vi "MEMR-Compute Noise Floor (single traces).vi"(0 "State In":T2, 5 "Analysis":T1, 7 "Avg":dbl[][](array[numeric]), 9 "Navg":i32, 11 "N":i32=1000) -> (4 "Noise spectra":cluster{"Freq (Hz)":dbl[], "Mag (dB)":dbl[]}[](array[cluster]))   [LabVIEW 2020]
uses:
  Typedefs/MEMR-Analysis State.ctl
  MEMR-Offline Analysis Parameters.ctl
  Typedefs/MEMR-Analysis.ctl
  PXI DAQ VIs/Utility VIs/Array Dimensions (2D).vi
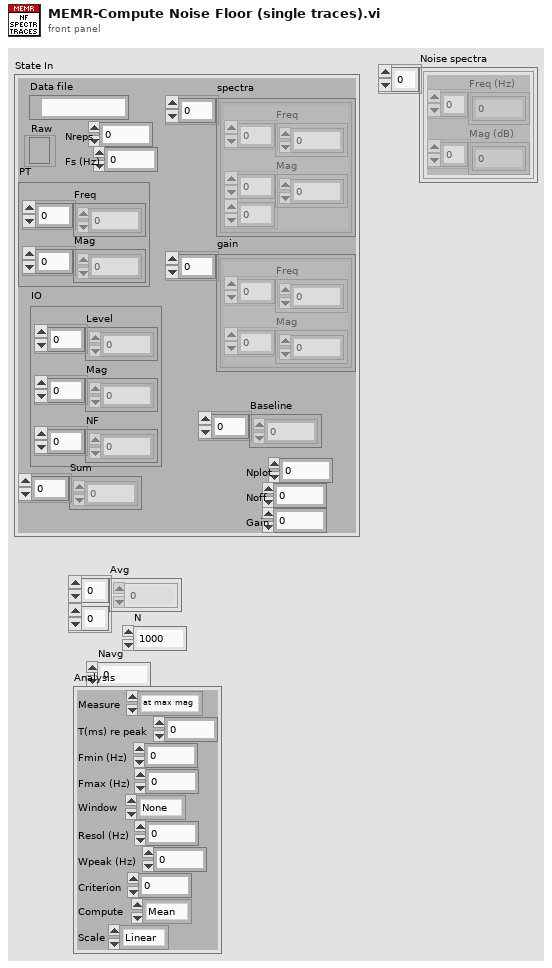
[diagram p1: front panel]
types:
  T1 = typedef "MEMR-Offline Analysis Parameters.ctl" = cluster{"Measure":enum16{"at max mag", "at max gain", "over window", "optimize", "Keefe"}, "T(ms) re peak":dbl, "Fmin (Hz)":dbl, "Fmax (Hz)":dbl, "Window":enum16{"None", "Hanning", "Hamming"}, "Resol (Hz)":dbl, "Wpeak (Hz)":dbl, "Criterion":dbl, "Compute":enum16{"Mean", "Sum"}, "Scale":enum16{"Linear", "Log"}}
  T2 = typedef "MEMR-Analysis State.ctl" = cluster{"Data file":path, "Raw":refnum<file>, "PT":cluster{"Freq":dbl[], "Mag":dbl[]}, "IO":cluster{"Level":dbl[], "Mag":dbl[], "NF":dbl[]}, "Nreps":i32, "Fs (Hz)":dbl, "Sum":dbl[], "Nplot":i32, "Noff":i32, "Gain":dbl, "spectra":cluster{"Freq":dbl[], "Mag":dbl[][]}[], "gain":cluster{"Freq":dbl[], "Mag":dbl[]}[], "Baseline":dbl[]}
  T3 = typedef "MEMR-Analysis.ctl" = cluster{"T(ms) re peak":dbl, "Fmin (Hz)":dbl, "Fmax (Hz)":dbl, "Window":enum16{"None", "Hanning", "Hamming"}, "Gain (dB)":dbl, "Resol (Hz)":dbl}
  T4 = cluster{"Freq (Hz)":dbl[], "+Freq. Mag of FFT (dB rms)":dbl[]}
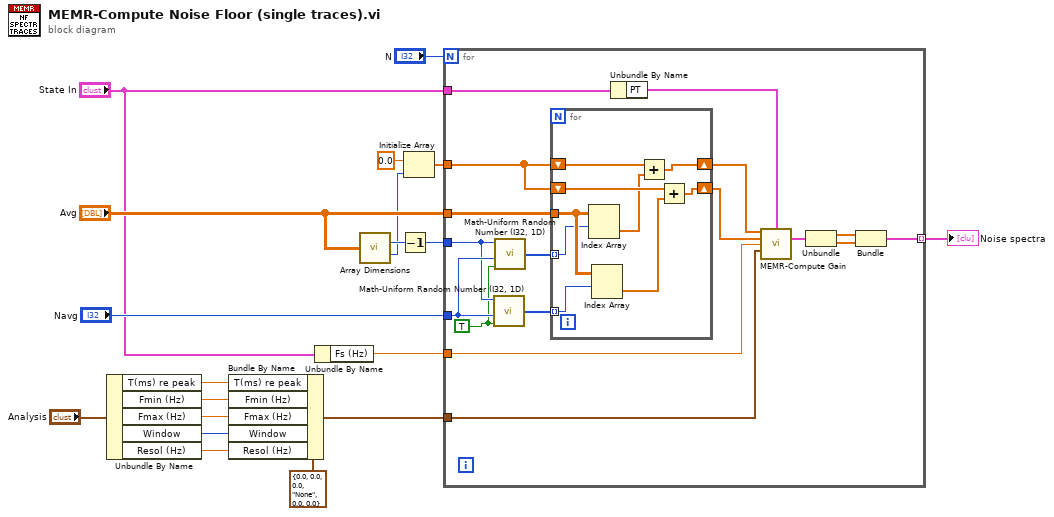
[diagram p0: block diagram]
diagram:
  n1 = Unbundle By Name("Analysis") -> ("T(ms) re peak"=w12:dbl, "Fmin (Hz)"=w11:dbl, "Fmax (Hz)"=w10:dbl, "Window"=w9:enum16{"None", "Hanning", "Hamming"}, "Resol (Hz)"=w8:dbl)
  n2 = Bundle By Name(cluster=T3 {"T(ms) re peak"=0.0, "Fmin (Hz)"=0.0, "Fmax (Hz)"=0.0, "Window"=enum."None", "Gain (dB)"=0.0, "Resol (Hz)"=0.0} ("Analysis"), "T(ms) re peak"=w12, "Fmin (Hz)"=w11, "Fmax (Hz)"=w10, "Window"=w9, "Resol (Hz)"=w8) -> (w7:T3)
  n3 = Unbundle By Name("State In") -> ("Fs (Hz)"=w16:dbl)
  n4 = call-poly "Array Dimensions.vi"("2D Array"="Avg") -> ("# rows"=w5:i32, "# columns"=w3:i32)  [unwired: 13 in]
  n5 = Decrement(x=w5) -> (x-1=w4:i32)
  n6 = Initialize Array(0.0 ("element"), w3) -> (w1:dbl[])
  n7 = for {
    N: "N" -> [_]
    tunnel: "State In" -> [w36]
    tunnel: "Avg" -> [w35]
    tunnel: w7 -> [w34]
    tunnel: "Navg" -> [w27]
    tunnel: w16 -> [w33]
    tunnel: [w32] -> w15 mode=indexing
    tunnel: w4 -> [w26]
    tunnel: w1 -> [w22]
    w25 = TRUE ("Replace?")
    n8 = call "Math-Uniform Random Number (I32, 1D).vi"("Replace?"=w25, "N"=w27, "Ymax"=w26) -> ("Random Ints"=w24:i32[])  [unwired: 3 in]
    n9 = call "Math-Uniform Random Number (I32, 1D).vi"("Replace?"=w25, "N"=w27, "Ymax"=w26) -> ("Random Ints"=w23:i32[])  [unwired: 3 in]
    n10 = for {
      tunnel: w35 -> [w45]
      tunnel: w24 -> [w43] mode=indexing
      tunnel: w23 -> [w44] mode=indexing
      shift-right: [w40] -> w21
      shift-left: w22 -> [w42]
      shift-right: [w38] -> w20
      shift-left: w22 -> [w41]
      n11 = Index Array(array=w45, index (row)=w44) -> (element=w39:dbl[])  [unwired: 1 in]
      n12 = Index Array(array=w45, index (row)=w43) -> (element=w37:dbl[])  [unwired: 1 in]
      n13 = Add(x=w42, y=w39) -> (x+y=w40:dbl[])
      n14 = Add(x=w41, y=w37) -> (x+y=w38:dbl[])
    }
    n15 = Unbundle By Name(w36) -> ("PT"=w31:cluster{"Freq":dbl[], "Mag":dbl[]})
    n16 = call "MEMR-Compute Gain.vi"("Test"=w21, "PT"=w31, "Baseline"=w20, "Fs (Hz)"=w33, "Analysis"=w34) -> ("gain spectrum"=w30:T4)  [unwired: 8 in, 2 out]
    n17 = Unbundle(w30) -> ("Freq (Hz)"=w29:dbl[], "+Freq. Mag of FFT (dB rms)"=w28:dbl[])
    n18 = Bundle("Freq (Hz)"=w29, "+Freq. Mag of FFT (dB rms)"=w28) -> (w32:T4)  [unwired: 1 in]
  }
  "Noise spectra" <- w15
